vi "Make_photon_buffers.vi"(10 "Array 3":u64[](array[numeric]), 11 "Array 4":u64[][](array[numeric])) -> (2 "Array":u64[][](array[numeric]), 3 "Array 2":u64[][](array[numeric]))   [LabVIEW 2023]
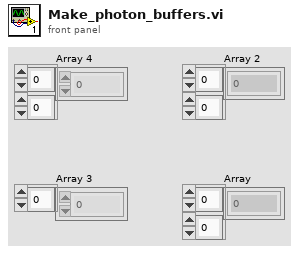
[diagram p1: front panel]
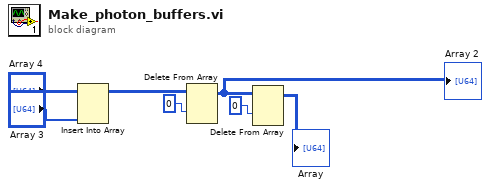
[diagram p0: block diagram]
diagram:
  n1 = Insert Into Array(array="Array 4", new element="Array 3") -> (w4:u64[][])  [unwired: 2 in]
  n2 = Delete From Array(array=w4, index (row)=0) -> (array with subset deleted=w6:u64[][])  [unwired: 2 in, 1 out]
  "Array 2" <- w6
  n3 = Delete From Array(array=w6, index (row)=0) -> (array with subset deleted=→"Array":u64[][])  [unwired: 2 in, 1 out]
